vi "rolling_digit.vi"(4 "Position":cluster{"left":i16, "top":i16}={"left"=40, "top"=22}, 5 "Background color":u32(colorbox)=14803425, 7 "value":dbl(slide)=2.0 scale=9.0..11.0, 10 "pict in":picture) -> (3 "pict out":picture)   [LabVIEW 2017]
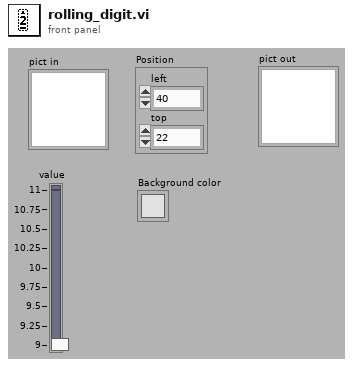
[diagram p1: front panel]
types:
  T1 = cluster{"left":i16, "top":i16, "right":i16, "bottom":i16}
  T2 = cluster{"Width":i16, "Style":enum32{"Solid", "Dash", "Dot", "DashDot", "DashDotDot"}}
  T3 = enum16{"User-specified Font", "Application Font", "System Font", "Dialog Font"}
  T4 = cluster{"Font Name:":string, "Size":i16, "Strikeout?":bool, "Italic?":bool, "Underline?":bool, "Outline?":bool, "Shadow?":bool, "Bold?":bool}
  T5 = typedef "imagedata.ctl" = cluster{"image type":i32, "image depth":i32, "image":u8[], "mask":u8[], "colors":u32[], "Rectangle":cluster{"left":i16, "top":i16, "right":i16, "bottom":i16}}
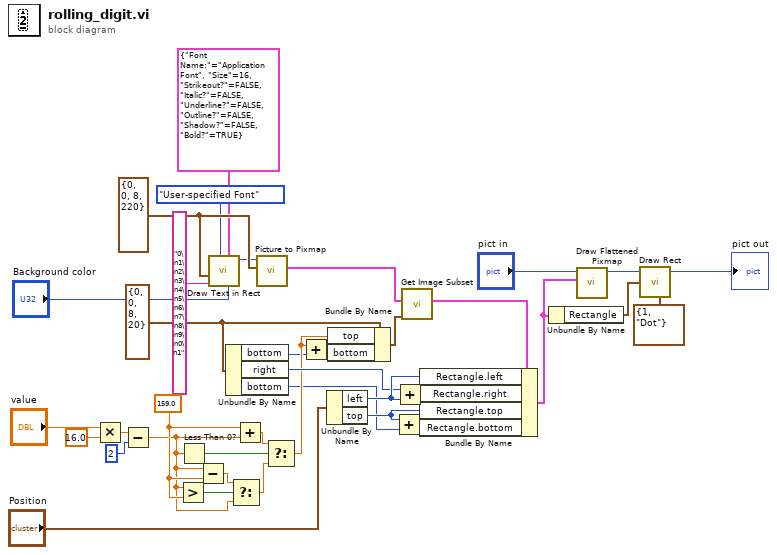
[diagram p0: block diagram]
diagram:
  w30 = 159.0 ("x 2")
  w14 = T1 {"left"=0, "top"=0, "right"=8, "bottom"=20} ("rect 2")
  w12 = T1 {"left"=0, "top"=0, "right"=8, "bottom"=220} ("rect")
  n1 = Multiply(x="value", y=16.0) -> (x*y=w21:dbl)
  n2 = Subtract(x=w21, y=2) -> (x-y=w28:dbl)
  n3 = Greater?(x=w28, y=w30) -> (0:w27:bool)
  n4 = Less Than 0?(x=w28) -> (x < 0?=w24:bool)
  n5 = Subtract(x=w28, y=w30) -> (x-y=w26:dbl)
  n6 = call <vilib>:"Draw Text in Rect.vi"("BG color(transparent)"="Background color", "[user-specified font]"=T4 {"Font Name:"="Application Font", "Size"=16, "Strikeout?"=FALSE, "Italic?"=FALSE, "Underline?"=FALSE, "Outline?"=FALSE, "Shadow?"=FALSE, "Bold?"=TRUE}, "desired font(Application)"=T3."User-specified Font", "text"="0\n1\n2\n3\n4\n5\n6\n7\n8\n9\n0\n1", "rect"=w12) -> ("new picture"=w8:picture)  [unwired: 6 in]
  n7 = Unbundle By Name(w14) -> ("bottom"=w13:i16, "right"=w34:i16, "bottom"=w3:i16)
  n8 = Select(t=w26, s=w27, f=w28) -> (s? t:f=w31:dbl)
  n9 = Add(x=w30, y=w28) -> (x+y=w25:dbl)
  n10 = call <vilib>:"Picture to Pixmap.vi"("rect"=w12, "picture"=w8) -> ("image data"=w4:T5)  [unwired: 8 in, 1 out]
  n11 = Select(t=w25, s=w24, f=w31) -> (s? t:f=w29:dbl)
  n12 = Add(x=w29, y=w13) -> (x+y=w9:dbl)
  n13 = Unbundle By Name("Position") -> ("left"=w35:i16, "top"=w33:i16)
  n14 = Bundle By Name(cluster=w14, "top"=w29, "bottom"=w9) -> (w10:T1)
  n15 = Add(x=w33, y=w3) -> (x+y=w20:i16)
  n16 = Add(x=w34, y=w35) -> (x+y=w11:i16)
  n17 = call <vilib>:"Get Image Subset.vi"("subset rect"=w10, "image data"=w4) -> ("image subset"=w15:T5)  [unwired: 4 in, 1 out]
  n18 = Bundle By Name(cluster=w15, "Rectangle.left"=w35, "Rectangle.right"=w11, "Rectangle.top"=w33, "Rectangle.bottom"=w20) -> (w16:T5)
  n19 = Unbundle By Name(w16) -> ("Rectangle"=w36:T1)
  n20 = call <vilib>:"Draw Flattened Pixmap.vi"("image data"=w16, "picture"="pict in") -> ("new picture"=w17:picture)  [unwired: 7 in]
  n21 = call <vilib>:"Draw Rect.vi"("picture"=w17, "rect"=w36, "pen"=T2 {"Width"=1, "Style"=enum."Dot"}) -> ("new picture"=→"pict out":picture)  [unwired: 6 in]
